vi "Insert into array.vi"() -> ()   [LabVIEW 2014]
panel:
  out "output array":i32[](array[numeric])
  in  "Array":i32[](array[numeric])
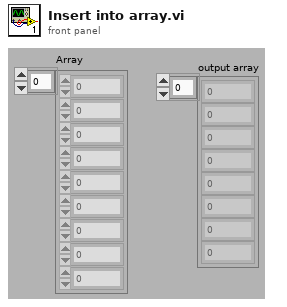
[diagram p1: front panel]
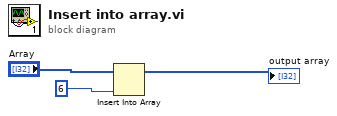
[diagram p0: block diagram]
diagram:
  n1 = Insert Into Array(array="Array", new element=6 ("new element/subarray")) -> (→"output array":i32[])  [unwired: 1 in]
